vi "ImageMagic Label Wrapper.vi"(4 "Font":T1={"Font Name"="Tahoma", "Size"=20, "Strikeout?"=FALSE, "Italic?"=TRUE, "Underline?"=TRUE, "Bold?"=FALSE}, 6 "Label Position":T2, 8 "error in (no error)":errorcluster, 9 "Text":string, 10 "Output File":path, 11 "Input File":path) -> (0 "error out":errorcluster)   [LabVIEW 2020, in "VIDiffImageMagic.lvlib"]
uses:
  VIDiffImageMagic.lvlib
  Label Position.ctl
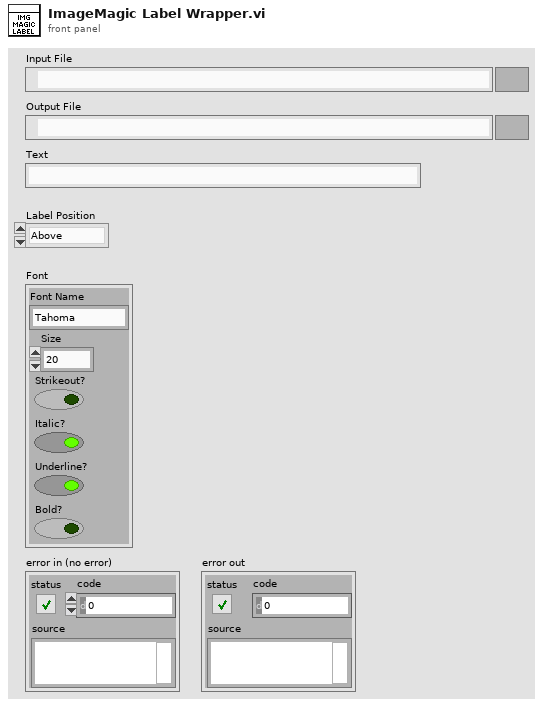
[diagram p1: front panel]
types:
  T1 = cluster{"Font Name":string, "Size":i16, "Strikeout?":bool, "Italic?":bool, "Underline?":bool, "Bold?":bool}
  T2 = typedef "VIDiffImageMagic.lvlib/Label Position.ctl" = enum16{"Above", "Below"}
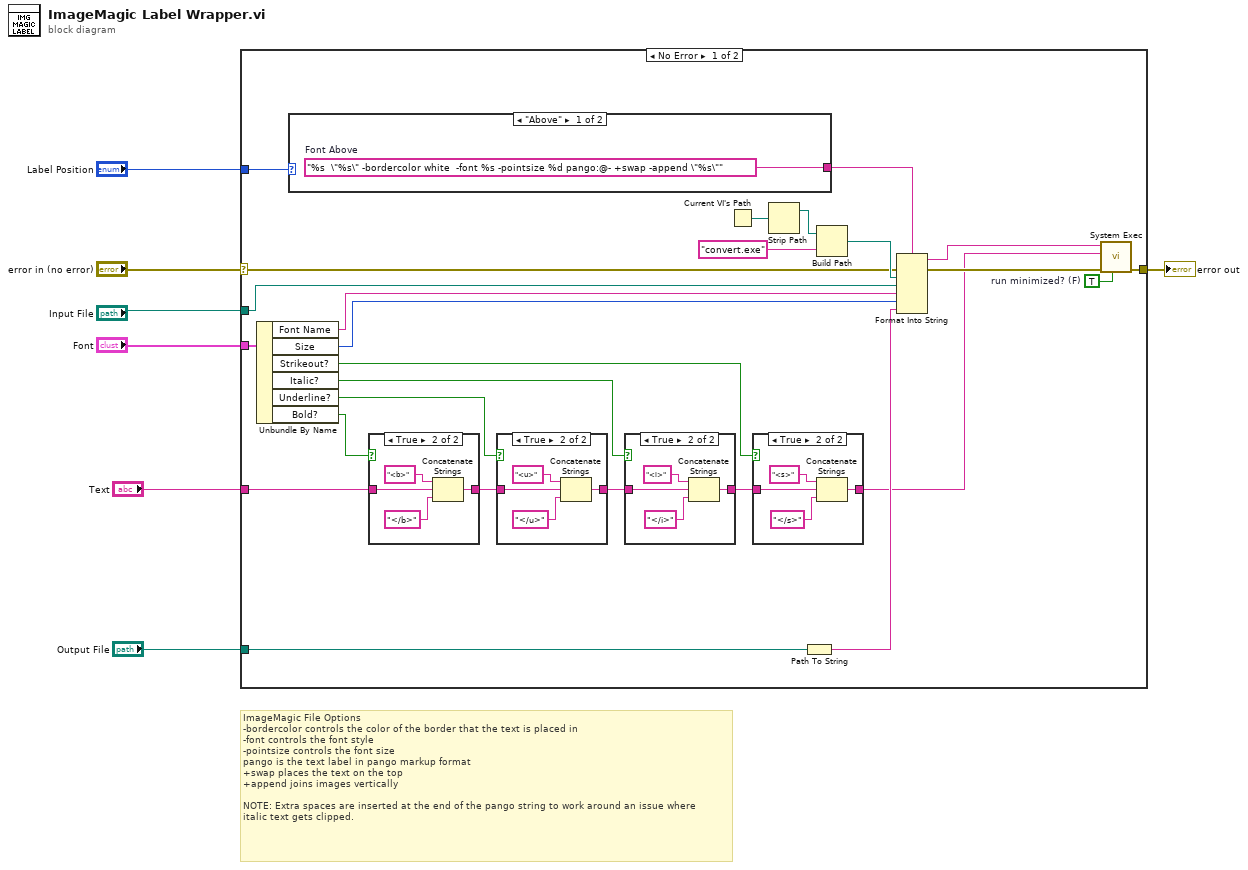
[diagram p0: block diagram]
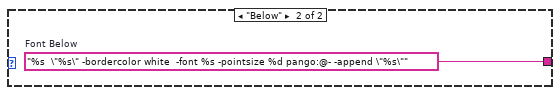
[diagram p6: hidden frame]
diagram:
  # "ImageMagic File Options\n-bordercolor controls the color of the border that the text is placed in\n-font controls the font style\n-pointsize controls the font size\npango is the text label in pango markup format\n+swap places the text on the top\n+append joins images vertically\n\nNOTE: Extra spaces are inserted at the end of the pango string to work around an issue where\nitalic text gets clipped."
  n1 = case shown="No Error" "error in (no error)" {
    selector: "error in (no error)" -> [w24 w56]
    tunnel: [w29 w56] -> w7
    tunnel: "Output File" -> [w26 _]
    tunnel: "Input File" -> [w20 _]
    tunnel: "Label Position" -> [w23 _]
    tunnel: "Font" -> [w19 _]
    tunnel: "Text" -> [w13 _]
    frame No Error {
      w31 = TRUE  # run minimized? (F)
      n2 = Unbundle By Name(w19) -> ("Font Name"=w18:string, "Size"=w17:i16, "Strikeout?"=w9:bool, "Italic?"=w10:bool, "Underline?"=w11:bool, "Bold?"=w12:bool)
      n3 = case shown="\"Above\"" w23 {
        tunnel: [w54 w55] -> w25
        frame "Above" {
          w54 = "%s  \"%s\" -bordercolor white  -font %s -pointsize %d pango:@- +swap -append \"%s\""  # Font Above
        }
        frame "Below" {
          w55 = "%s  \"%s\" -bordercolor white  -font %s -pointsize %d pango:@- -append \"%s\""  # Font Below
        }
      }
      n4 = case shown="True" w12 {
        tunnel: [w49 w51] -> w16
        tunnel: w13 -> [w49 w50]
        frame False {
        }
        frame True {
          n5 = Concatenate Strings("<b>" ("string"), w50, "</b>" ("string")) -> (w51:string)
        }
      }
      n6 = case shown="True" w11 {
        tunnel: [w44 w46] -> w15
        tunnel: w16 -> [w44 w45]
        frame False {
        }
        frame True {
          n7 = Concatenate Strings("<u>" ("string"), w45, "</u>" ("string")) -> (w46:string)
        }
      }
      n8 = case shown="True" w10 {
        tunnel: [w39 w41] -> w14
        tunnel: w15 -> [w39 w40]
        frame False {
        }
        frame True {
          n9 = Concatenate Strings("<i>" ("string"), w40, "</i>" ("string")) -> (w41:string)
        }
      }
      n10 = Current VI's Path() -> (path=w22:path)
      n11 = case shown="True" w9 {
        tunnel: [w34 w36] -> w8
        tunnel: w14 -> [w34 w35]
        frame False {
        }
        frame True {
          n12 = Concatenate Strings("<s>" ("string"), w35, "</s>" ("string")) -> (w36:string)
        }
      }
      n13 = Strip Path(path=w22) -> (stripped path=w21:path)  [unwired: 1 out]
      n14 = Path To String(path=w26) -> (string=w27:string)
      n15 = Build Path(base path=w21, name or relative path="convert.exe") -> (appended path=w33:path)
      n16 = Format Into String(format string=w25, error in=w24, w33, w20, w18, w17, w27) -> (resulting string=w30:string, error out=w28:errorcluster)  [unwired: 1 in]
      n17 = call <vilib>:"System Exec.vi"("run minimized? (F)"=w31, "error in (no error)"=w28, "standard input"=w8, "command line"=w30) -> ("error out"=w29:errorcluster)  [unwired: 4 in, 3 out]
    }
    frame Error {
    }
  }
  "error out" <- w7
